vi "Velocidad_rpm.vi"(10 "data":dynamicdata(waveform), 11 "Numeric in":dbl) -> (3 "Numeric out":dbl)   [LabVIEW 2019]
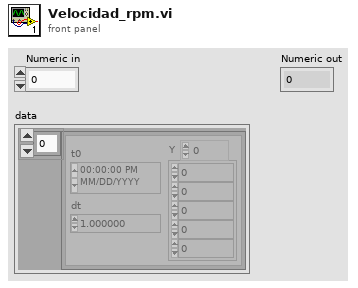
[diagram p1: front panel]
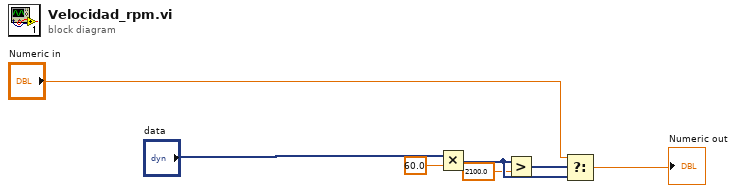
[diagram p0: block diagram]
diagram:
  n1 = Multiply(x="data", y=60.0) -> (x*y=w4:dynamicdata)
  n2 = Greater?(x=w4, y=2100.0) -> (0:w3:dynamicdata)
  n3 = Select(t="Numeric in", s=w3, f=w4) -> (s? t:f=→"Numeric out":dbl)
